vi "Test_Count.vi"(8 "error in (no error)":errorcluster, 11 "TestCase in":refnum<class "ListImp_Functional.lvclass">) -> (0 "error out":errorcluster, 3 "TestCase out":refnum<class "ListImp_Functional.lvclass">)   [LabVIEW 2009, in "ListImp_Functional.lvclass"]
uses:
  ListImp_Functional.lvclass
  ListImp_Functional.lvclass/ListImp_Functional.ctl
  source/Lists/List/List.lvclass
  UnitTestComparisons/UnitTestComparisons.lvlib
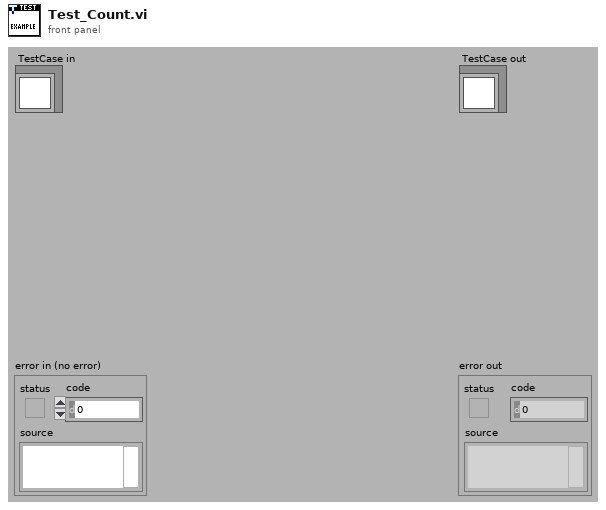
[diagram p1: front panel]
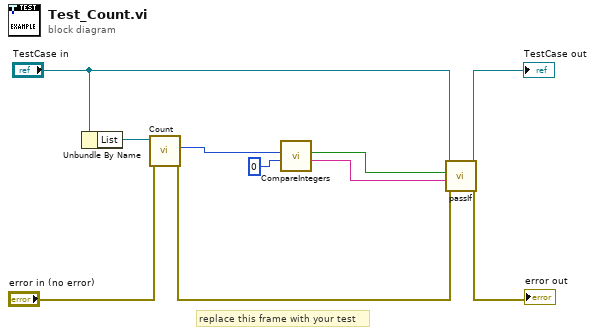
[diagram p0: block diagram]
diagram:
  # "replace this frame with your test"
  n1 = Unbundle By Name("TestCase in") -> ("List"=w7:refnum<class "List.lvclass">)
  n2 = call-dynamic "Count.vi"("error in (no error)"="error in (no error)", "List in"=w7) -> ("error out"=w5:errorcluster, "Number of Items"=w4:i32)  [unwired: 7 in, 1 out]
  n3 = call "CompareIntegers.vi"("Expected Value"=0, "Actual Value"=w4) -> ("Message"=w2:string, "Equal?"=w3:bool)  [unwired: 8 in]
  n4 = call-dynamic "passIf.vi"("error in (no error)"=w5, "message (\"\")"=w2, "pass"=w3, "TestCase in"="TestCase in") -> ("error out"=→"error out":errorcluster, "TestCase out"=→"TestCase out":refnum<class "ListImp_Functional.lvclass">)  [unwired: 6 in]
